vi "Teleop.vi"(10 "Match Info":T1={"Autonomous Elapsed Seconds"=0.0, "TeleOp Elapsed Seconds"=0.0, "Disabled Elapsed Seconds"=0.0, "Visited Autonomous"=FALSE, "Visited TeleOp"=FALSE, "Visited Disabled"=FALSE, "Autonomous Settings"={"Autonomous Style"=enum."Independent", "VI Refnum"=refnum}}, 11 "Call Context":T2) -> ()   [LabVIEW 2020]
doc: "This VI is called for each TeleOp packet received from the DS where the robot is not disabled. It is often used to read from the joysticks and update I/O or to update setpoints for timed control loops. It should complete and return within 20 milliseconds or it may miss DS packets."
uses:
  <vilib>/Rock Robotics/WPI/DriverStation/WPI_DriverStationDerivedRobotMode.ctl
  <vilib>/Rock Robotics/WPI/DriverStation/WPI_DriverStationMatch Info.ctl
  <vilib>/Rock Robotics/WPI/Utilities/WPI_GetSetVariantRefNum.vi
  Robot Global Data.vi
  <vilib>/Rock Robotics/Network Tables/NT Write Boolean Array.vi
  <vilib>/Rock Robotics/Network Tables/NT Write Numeric Array.vi
panel:
  out "Left Rumble":sgl
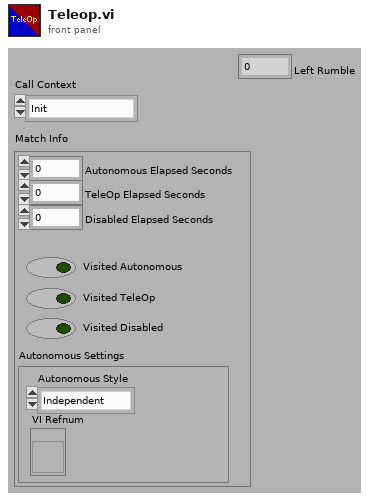
[diagram p1: front panel]
types:
  T1 = typedef "WPI_DriverStationMatch Info.ctl" = cluster{"Autonomous Elapsed Seconds":dbl, "TeleOp Elapsed Seconds":dbl, "Disabled Elapsed Seconds":dbl, "Visited Autonomous":bool, "Visited TeleOp":bool, "Visited Disabled":bool, "Autonomous Settings":cluster{"Autonomous Style":enum16{"Iterative", "Independent"}, "VI Refnum":refnum<vi>}}
  T2 = typedef "WPI_DriverStationDerivedRobotMode.ctl" = enum16{"Init", "Execute", "Stop"}
  T3 = typedef "WPI_JoystickDevRef.ctl" = cluster{"Device":T4}
  T4 = typedef "WPI_JoystickDeviceEnum.ctl" = enum16{"USB 0", "USB 1", "USB 2", "USB 3", "USB 4", "USB 5"}
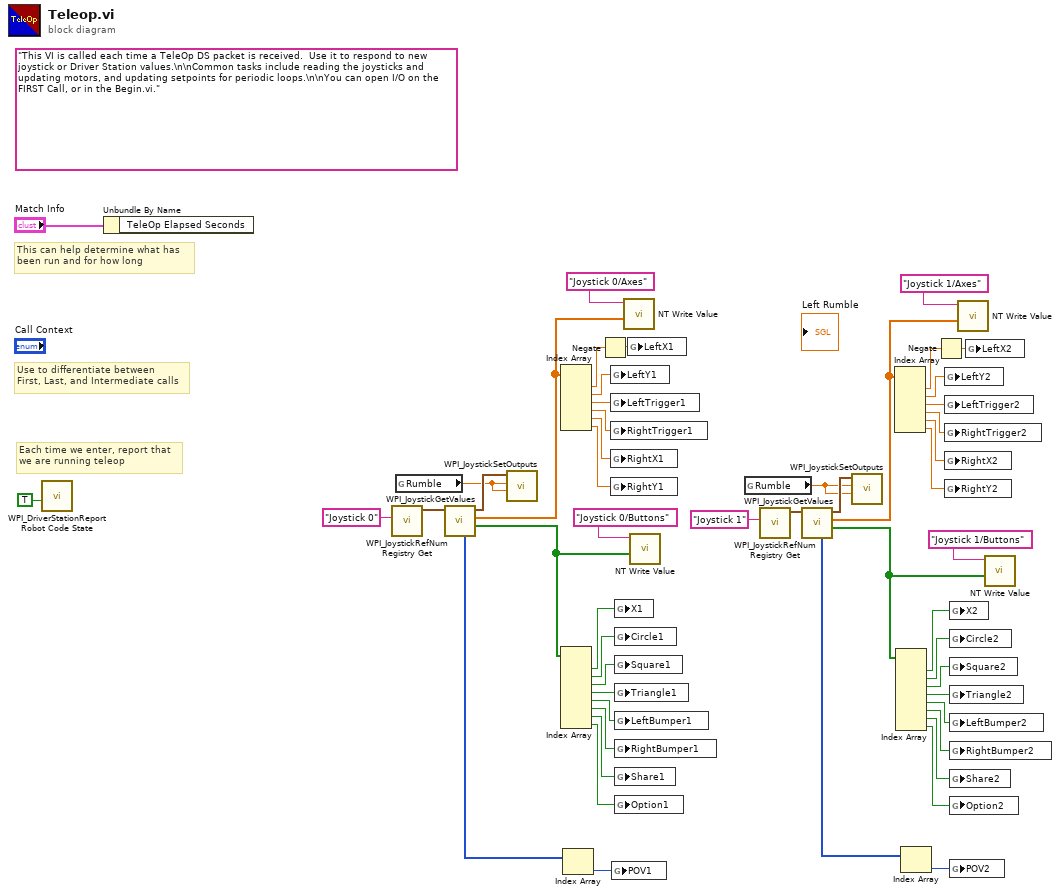
[diagram p0: block diagram]
diagram:
  (unwired) "This VI is called each time a TeleOp DS packet is received.  Use it to respond to new joystick or Driver Station values.\n\nCommon tasks include reading the joysticks and updating motors, and updating setpoints for periodic loops.\n\nYou can open I/O on the FIRST Call, or in the Begin.vi."
  # "Each time we enter, report that\nwe are running teleop"
  # "Use to differentiate between\nFirst, Last, and Intermediate calls"
  # "This can help determine what has\nbeen run and for how long"
  n1 = call <vilib>:"WPI_DriverStationReport Robot Code State.vi"("TeleOp"=TRUE ("Autonomous")) -> ()  [unwired: 10 in, 1 out]
  n2 = Unbundle By Name("Match Info") -> ()  [unwired: 1 out]
  n3 = call <vilib>:"WPI_JoystickRefNum Registry Get.vi"("refnum name"="Joystick 0") -> ("JoystickDevRef"=w50:T3)  [unwired: 1 in, 9 out]
  n4 = global read "Robot Global Data.vi" "Rumble"() -> (w2:sgl)
  n5 = call <vilib>:"WPI_JoystickGetValues.vi"("JoystickDevRef"=w50) -> ("Buttons"=w45:bool[], "Axes"=w46:dbl[], "JoystickDevRef"=w4:T3, "POVs"=w9:i16[])  [unwired: 6 in, 1 out]
  n6 = call <vilib>:"WPI_JoystickSetOutputs.vi"("Right Rumble"=w2, "Left Rumble"=w2, "JoystickDevRef"=w4) -> ()  [unwired: 7 in, 2 out]
  n7 = Index Array(array=w46) -> (element #1=w38:dbl, element #2=w37:dbl, element #3=w36:dbl, element #4=w35:dbl, element #5=w34:dbl, element #6=w33:dbl)  [unwired: 6 in]
  n8 = Index Array(array=w45) -> (element #1=w44:bool, element #2=w43:bool, element #3=w42:bool, element #4=w41:bool, element #5=w40:bool, element #6=w39:bool, element #7=w14:bool, element #8=w13:bool)  [unwired: 8 in]
  n9 = Index Array(array=w9) -> (element=w8:i16)  [unwired: 1 in]
  n10 = Negate(x=w38) -> (-x=w10:dbl)
  n11 = global write "Robot Global Data.vi" "LeftY1"(w37) -> ()
  n12 = global write "Robot Global Data.vi" "LeftTrigger1"(w36) -> ()
  n13 = global write "Robot Global Data.vi" "RightTrigger1"(w35) -> ()
  n14 = global write "Robot Global Data.vi" "RightX1"(w34) -> ()
  n15 = global write "Robot Global Data.vi" "RightY1"(w33) -> ()
  n16 = global write "Robot Global Data.vi" "POV1"(w8) -> ()
  n17 = global write "Robot Global Data.vi" "X1"(w44) -> ()
  n18 = global write "Robot Global Data.vi" "Circle1"(w43) -> ()
  n19 = global write "Robot Global Data.vi" "Square1"(w42) -> ()
  n20 = global write "Robot Global Data.vi" "Triangle1"(w41) -> ()
  n21 = global write "Robot Global Data.vi" "LeftBumper1"(w40) -> ()
  n22 = global write "Robot Global Data.vi" "RightBumper1"(w39) -> ()
  n23 = global write "Robot Global Data.vi" "Share1"(w14) -> ()
  n24 = global write "Robot Global Data.vi" "Option1"(w13) -> ()
  n25 = call-poly <vilib>:"NT Write Value.vi"("Numeric Array"=w46, "Name"="Joystick 0/Axes") -> ()  [unwired: 9 in, 1 out]
  n26 = global write "Robot Global Data.vi" "LeftX1"(w10) -> ()
  n27 = call-poly <vilib>:"NT Write Value.vi"("Boolean Array"=w45, "Name"="Joystick 0/Buttons") -> ()  [unwired: 9 in, 1 out]
  n28 = global read "Robot Global Data.vi" "Rumble"() -> (w1:sgl)
  n29 = call <vilib>:"WPI_JoystickRefNum Registry Get.vi"("refnum name"="Joystick 1") -> ("JoystickDevRef"=w16:T3)  [unwired: 1 in, 9 out]
  n30 = call <vilib>:"WPI_JoystickGetValues.vi"("JoystickDevRef"=w16) -> ("Buttons"=w20:bool[], "Axes"=w19:dbl[], "JoystickDevRef"=w3:T3, "POVs"=w6:i16[])  [unwired: 6 in, 1 out]
  n31 = call <vilib>:"WPI_JoystickSetOutputs.vi"("Right Rumble"=w1, "Left Rumble"=w1, "JoystickDevRef"=w3) -> ()  [unwired: 7 in, 2 out]
  n32 = Index Array(array=w19) -> (element #1=w27:dbl, element #2=w28:dbl, element #3=w29:dbl, element #4=w30:dbl, element #5=w31:dbl, element #6=w32:dbl)  [unwired: 6 in]
  n33 = Index Array(array=w20) -> (element #1=w21:bool, element #2=w22:bool, element #3=w23:bool, element #4=w24:bool, element #5=w25:bool, element #6=w26:bool, element #7=w12:bool, element #8=w11:bool)  [unwired: 8 in]
  n34 = Index Array(array=w6) -> (element=w7:i16)  [unwired: 1 in]
  n35 = Negate(x=w27) -> (-x=w5:dbl)
  n36 = global write "Robot Global Data.vi" "LeftY2"(w28) -> ()
  n37 = global write "Robot Global Data.vi" "LeftTrigger2"(w29) -> ()
  n38 = global write "Robot Global Data.vi" "RightTrigger2"(w30) -> ()
  n39 = global write "Robot Global Data.vi" "RightX2"(w31) -> ()
  n40 = global write "Robot Global Data.vi" "RightY2"(w32) -> ()
  n41 = global write "Robot Global Data.vi" "X2"(w21) -> ()
  n42 = global write "Robot Global Data.vi" "Circle2"(w22) -> ()
  n43 = global write "Robot Global Data.vi" "Square2"(w23) -> ()
  n44 = global write "Robot Global Data.vi" "Triangle2"(w24) -> ()
  n45 = global write "Robot Global Data.vi" "LeftBumper2"(w25) -> ()
  n46 = global write "Robot Global Data.vi" "RightBumper2"(w26) -> ()
  n47 = global write "Robot Global Data.vi" "Share2"(w12) -> ()
  n48 = global write "Robot Global Data.vi" "Option2"(w11) -> ()
  n49 = global write "Robot Global Data.vi" "POV2"(w7) -> ()
  n50 = call-poly <vilib>:"NT Write Value.vi"("Numeric Array"=w19, "Name"="Joystick 1/Axes") -> ()  [unwired: 9 in, 1 out]
  n51 = global write "Robot Global Data.vi" "LeftX2"(w5) -> ()
  n52 = call-poly <vilib>:"NT Write Value.vi"("Boolean Array"=w20, "Name"="Joystick 1/Buttons") -> ()  [unwired: 9 in, 1 out]
